vi "testRTDO.vi"() -> ()   [LabVIEW 2013]
panel:
  out "error out":errorcluster
  in  "DO0":bool
  in  "stop":bool
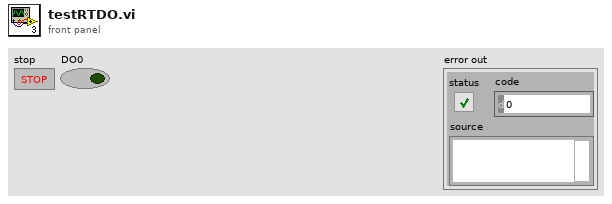
[diagram p1: front panel]
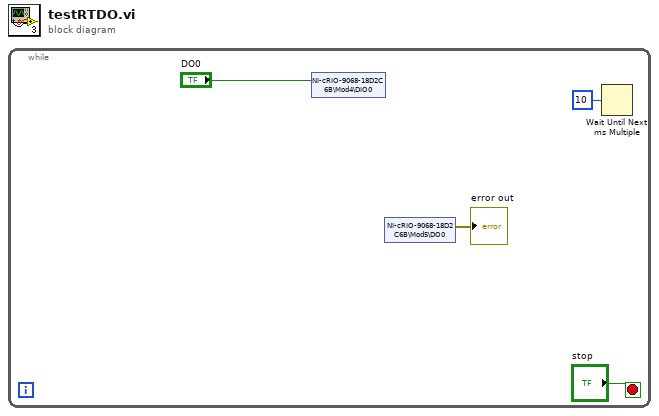
[diagram p0: block diagram]
diagram:
  n1 = while {
    stop <- "stop" stop-if-true
    n2 = shared-variable "NI-cRIO-9068-18D2C6B\\Mod4\\DIO0"("DO0") -> ()  [unwired: 1 in, 1 out]
    n3 = shared-variable "NI-cRIO-9068-18D2C6B\\Mod5\\DO0"() -> (error out=→"error out":errorcluster)  [unwired: 2 in]
    n4 = Wait Until Next ms Multiple(millisecond multiple=u32 10) -> ()  [unwired: 1 out]
  }
